vi "comm configure.vi"(5 "timeout (10000ms)":u32=10000, 6 "flow control":T2={"Flow Control"=0, "XOFF Character"=13, "XON Character"=11} {"Flow Control" items=["None"=0, "XON/XOFF"=1, "RTS/CTS"=2, "DTR/DSR"=4]}, 7 "termination settings":T1, 8 "error in (no error)":errorcluster, 9 "buffer size":cluster{"RX buffer":u32, "TX buffer":u32}={"RX buffer"=1024, "TX buffer"=1024}, 10 "serial settings":T3={"Baud Rate"=9600, "Data Bits"=8, "Parity"=0, "Stop Bits"=10} {"Stop Bits" items=["1.0"=10, "1.5"=15, "2.0"=20]; "Parity" items=["None", "Odd", "Even", "Mark", "Space"]}, 11 "Comm Handle":u64) -> (0 "error out":errorcluster, 3 "dup Comm Handle":u64)   [LabVIEW 2021, in "lvserial.lvlib"]
doc: "Initializes the serial port with the specified settings."
uses:
  lvserial.lvlib
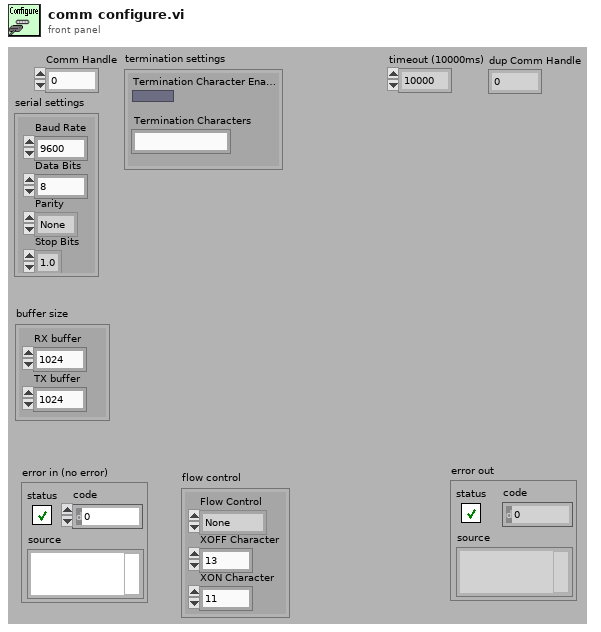
[diagram p1: front panel]
types:
  T1 = cluster{"Termination Character Enable":bool, "Termination Characters":string}
  T2 = cluster{"Flow Control":u16, "XOFF Character":u8, "XON Character":u8}
  T3 = cluster{"Baud Rate":u32, "Data Bits":u16, "Parity":u16, "Stop Bits":u16}
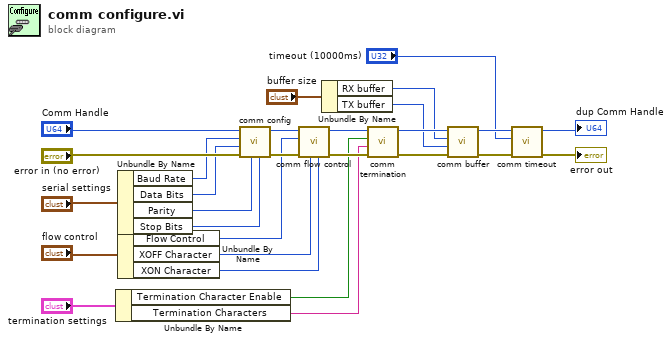
[diagram p0: block diagram]
diagram:
  n1 = Unbundle By Name("termination settings") -> ("Termination Character Enable"=w11:bool, "Termination Characters"=w10:string)
  n2 = Unbundle By Name("serial settings") -> ("Baud Rate"=w22:u32, "Data Bits"=w21:u16, "Parity"=w20:u16, "Stop Bits"=w19:u16)
  n3 = Unbundle By Name("flow control") -> ("Flow Control"=w16:u16, "XOFF Character"=w15:u8, "XON Character"=w14:u8)
  n4 = call "comm config.vi"("Stop Bits"=w19, "Parity"=w20, "error in (no error)"="error in (no error)", "Data Bits"=w21, "Baud Rate"=w22, "Comm Handle"="Comm Handle") -> ("error out"=w18:errorcluster, "dup Comm Handle"=w17:u64)  [unwired: 4 out]
  n5 = call "comm flow control.vi"("XON Character"=w14, "XOFF Character"=w15, "error in (no error)"=w18, "Flow Control"=w16, "Comm Handle"=w17) -> ("error out"=w13:errorcluster, "dup Comm Handle"=w12:u64)  [unwired: 5 out]
  n6 = Unbundle By Name("buffer size") -> ("RX buffer"=w7:u32, "TX buffer"=w6:u32)
  n7 = call "comm termination.vi"("error in (no error)"=w13, "termination characters"=w10, "Termination Character Enable"=w11, "Comm Handle"=w12) -> ("error out"=w8:errorcluster, "dup Comm Handle"=w9:u64)  [unwired: 6 out]
  n8 = call "comm buffer.vi"("error in (no error)"=w8, "Out Queue Size"=w6, "In Queue Size"=w7, "Comm Handle"=w9) -> ("error out"=w5:errorcluster, "dup Comm Handle"=w4:u64)  [unwired: 6 out]
  n9 = call "comm timeout.vi"("error in (no error)"=w5, "Timeout"="timeout (10000ms)", "Comm Handle"=w4) -> ("error out"=→"error out":errorcluster, "dup Comm Handle"=→"dup Comm Handle":u64)  [unwired: 7 out]
